vi "SubVI_Acc_Result.vi"(8 "error in (no error)":errorcluster caption="에러 입력(에러 없음)", 9 "Acc. duration pecent [%]":u16, 10 "Acc. index":i32, 11 "Filltered Acc Data":dbl[][](array[numeric])) -> (0 "error out":errorcluster caption="에러 출력", 1 "acc area":dbl format="%0.4f", 2 "acc Time":dbl, 3 "acc peak":dbl)   [LabVIEW 2013]
uses:
  <vilib>/Analysis/8numeric.llb/1D Numeric Integration.vi
  <vilib>/Analysis/NI_AALPro.lvlib
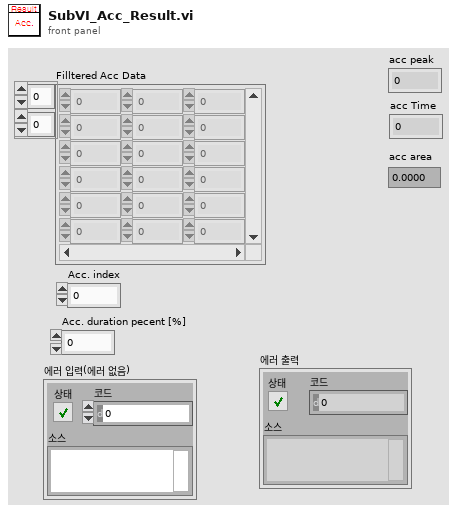
[diagram p1: front panel]
types:
  T1 = enum32{"Trapezoidal Rule", "Simpson's Rule", "Simpson's 3/8 Rule", "Bode Rule"}
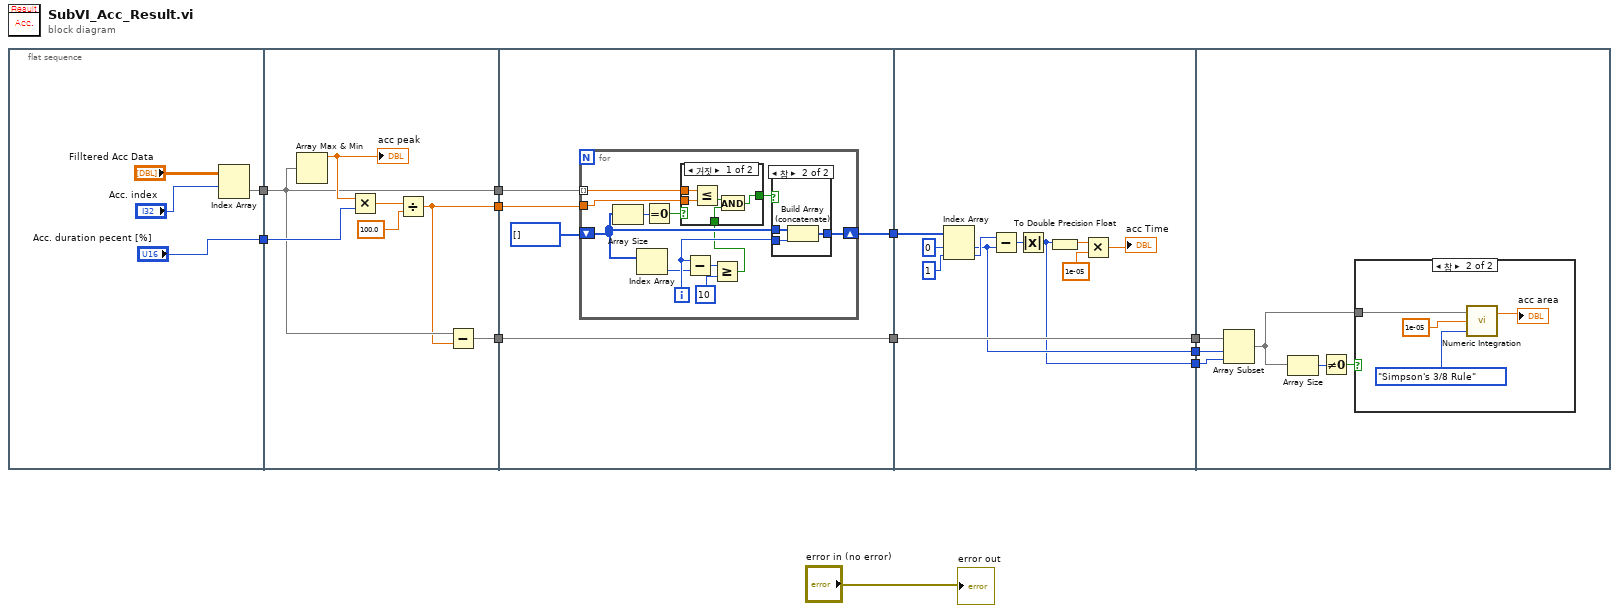
[diagram p0: block diagram]
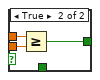
[diagram p2: hidden frame]
diagram:
  n1 = flat-sequence {
    tunnel: [w13] -> w11
    tunnel: ["Acc. duration pecent [%]"] -> w10
    tunnel: w11 -> [w18]
    tunnel: w10 -> [w20]
    tunnel: [w17] -> w9
    tunnel: [w18] -> w8
    tunnel: [w16] -> w7
    tunnel: w9 -> [w26]
    tunnel: w8 -> [w27]
    tunnel: w7 -> [w24]
    tunnel: [w25] -> w6
    tunnel: [w24] -> w4
    tunnel: w6 -> [w55]
    tunnel: [w54] -> w5
    tunnel: w4 -> [w54]
    tunnel: [w53] -> w3
    tunnel: [w52] -> w2
    tunnel: w5 -> [w65]
    tunnel: w3 -> [w64]
    tunnel: w2 -> [w63]
    frame #0 {
      n2 = Index Array(array="Filltered Acc Data", index (row)="Acc. index") -> (element=w13:dbl[])  [unwired: 1 in]
    }
    frame #1 {
      n3 = Array Max & Min(array=w18) -> (max value=w19:dbl)  [unwired: 3 out]
      "acc peak" <- w19
      n4 = Multiply(x=w19, y=w20) -> (x*y=w22:dbl)
      n5 = Divide(x=w22, y=100.0) -> (x/y=w17:dbl)
      n6 = Subtract(x=w18, y=w17) -> (x-y=w16:dbl[])
    }
    frame #2 {
      n7 = for {
        tunnel: w26 -> [w39]
        tunnel: w27 -> [w38] mode=indexing
        shift-right: [w36] -> w25
        shift-left: i32[] [] -> [w33]
        i -> [w32]
        n8 = Array Size(array=w33) -> (size(s)=w34:i32)
        n9 = Index Array(array=w33) -> (element=w31:i32)  [unwired: 1 in]
        n10 = Equal To 0?(x=w34) -> (x = 0?=w35:bool)
        n11 = Subtract(x=w32, y=w31) -> (x-y=w30:i32)
        n12 = Greater Or Equal?(x=w30, y=10) -> (x >= y?=w28:bool)
        n13 = case shown="거짓" w35 {
          tunnel: w39 -> [w43 w47]
          tunnel: w38 -> [w44 w46]
          tunnel: [w40 w45] -> w37
          tunnel: w28 -> [w42 _]
          frame False {
            n14 = Less Or Equal?(x=w44, y=w43) -> (x <= y?=w41:bool)
            n15 = And(x=w41, y=w42) -> (x .and. y?=w40:bool)
          }
          frame True {
            n16 = Greater Or Equal?(x=w46, y=w47) -> (x >= y?=w45:bool)
          }
        }
        n17 = case shown="참" w37 {
          tunnel: w32 -> [_ w51]
          tunnel: [w48 w50] -> w36
          tunnel: w33 -> [w48 w49]
          frame False {
          }
          frame True {
            n18 = Build Array (concatenate)(w49, w51) -> (w50:i32[])
          }
        }
      }
    }
    frame #3 {
      n19 = Index Array(array=w55, index #1=0 ("index"), index #2=1 ("index")) -> (element #1=w53:i32, element #2=w58:i32)
      n20 = Subtract(x=w58, y=w53) -> (x-y=w59:i32)
      n21 = Absolute Value(x=w59) -> (abs(x)=w52:i32)
      n22 = To Double Precision Float(number=w52) -> (double precision float=w60:dbl)
      n23 = Multiply(x=w60, y=1e-05) -> (x*y=→"acc Time":dbl)
    }
    frame #4 {
      n24 = Array Subset(array=w65, index=w64, length=w63) -> (w68:dbl[])
      n25 = Array Size(array=w68) -> (size(s)=w66:i32)
      n26 = Not Equal To 0?(x=w66) -> (x != 0?=w67:bool)
      n27 = case shown="참" w67 {
        tunnel: w68 -> [_ w70]
        frame False {
        }
        frame True {
          n28 = call-poly <vilib>:"Numeric Integration.vi"("integration method"=T1."Simpson's 3/8 Rule", "dt"=1e-05, "Input Array"=w70) -> ("result"=→"acc area":dbl)  [unwired: 1 out]
        }
      }
    }
  }
  "error out" <- "error in (no error)"
